vi "decode_serial_string.vi"(8 "Error In":errorcluster, 11 "Input Str":string) -> (0 "Error Out":errorcluster, 2 "Time":dbl, 3 "Current Values":T1)   [LabVIEW 2019]
doc: "Decode the serial string into its components."
uses:
  current_values_cluster_typedef.ctl
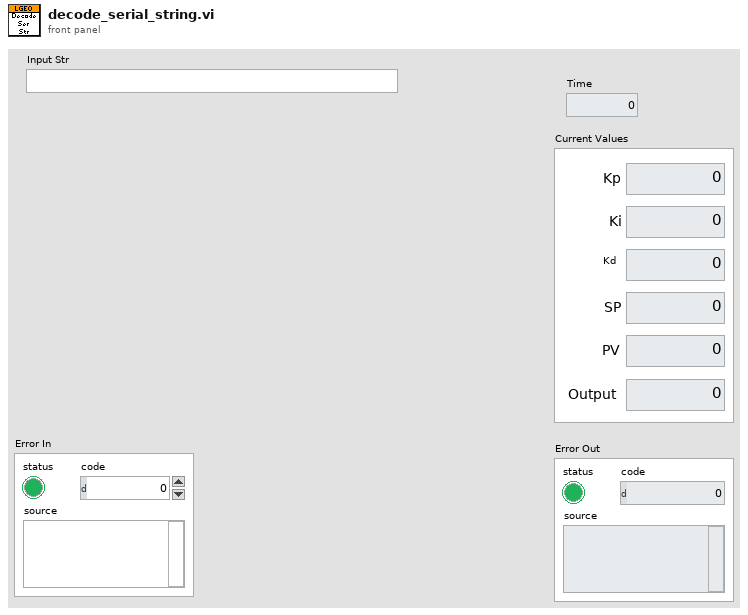
[diagram p1: front panel]
types:
  T1 = typedef "current_values_cluster_typedef.ctl" = cluster{"Kp":dbl, "Ki":dbl, "Kd":dbl, "SP":dbl, "PV":dbl, "Output":dbl}
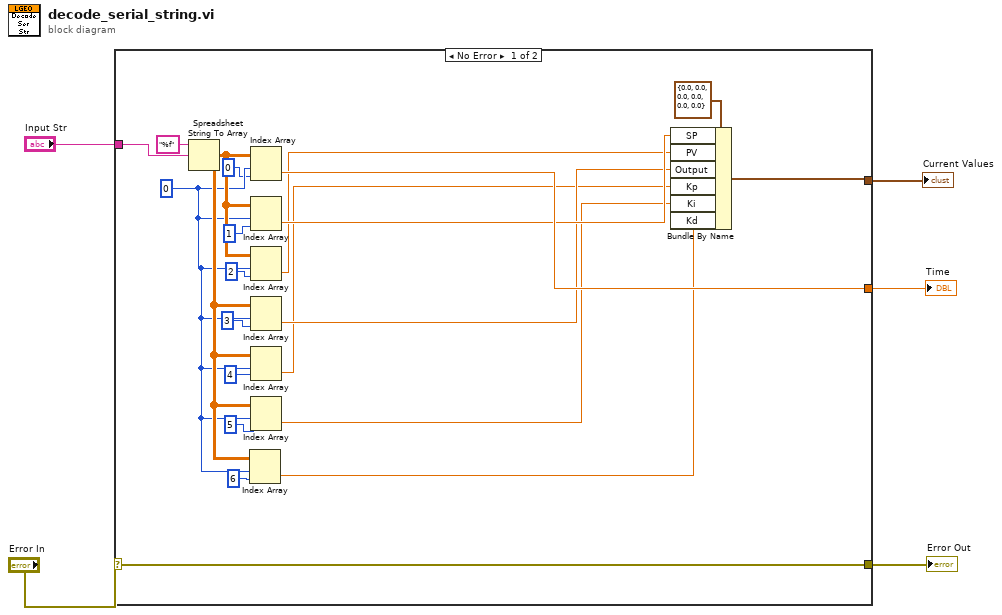
[diagram p0: block diagram]
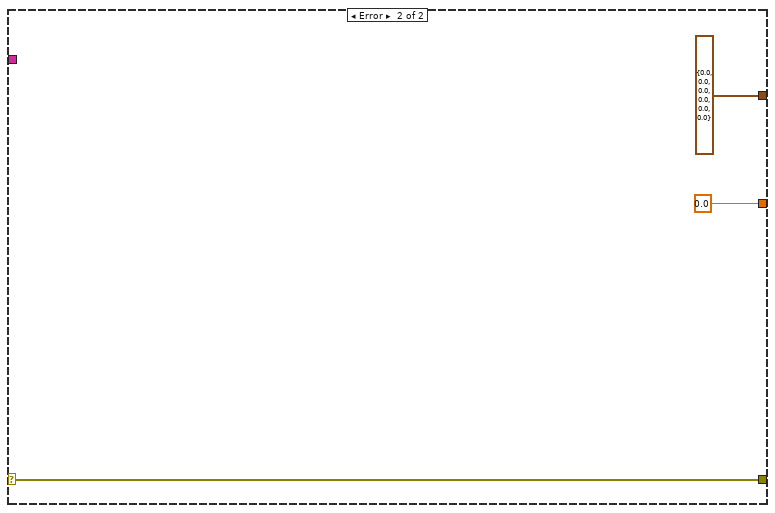
[diagram p2: hidden frame]
diagram:
  n1 = case shown="No Error" "Error In" {
    selector: "Error In" -> [w24 w29]
    tunnel: [w24 w29] -> w4
    tunnel: [w22 T1 {"Kp"=0.0, "Ki"=0.0, "Kd"=0.0, "SP"=0.0, "PV"=0.0, "Output"=0.0} ("Current Values")] -> w3
    tunnel: [w21 0.0 ("Time")] -> w2
    tunnel: "Input Str" -> [w26 _]
    frame No Error {
      w13 = 0
      n2 = Spreadsheet String To Array(format string="%f", spreadsheet string=w26) -> (array=w17:dbl[][])  [unwired: 2 in]
      n3 = Index Array(array=w17, index (row)=w13, index (col)=6) -> (element=w16:dbl)
      n4 = Index Array(array=w17, index (row)=w13, index (col)=0) -> (element=w21:dbl)
      n5 = Index Array(array=w17, index (row)=w13, index (col)=1) -> (element=w20:dbl)
      n6 = Index Array(array=w17, index (row)=w13, index (col)=2) -> (element=w19:dbl)
      n7 = Index Array(array=w17, index (row)=w13, index (col)=3) -> (element=w18:dbl)
      n8 = Index Array(array=w17, index (row)=w13, index (col)=4) -> (element=w14:dbl)
      n9 = Index Array(array=w17, index (row)=w13, index (col)=5) -> (element=w15:dbl)
      n10 = Bundle By Name(cluster=T1 {"Kp"=0.0, "Ki"=0.0, "Kd"=0.0, "SP"=0.0, "PV"=0.0, "Output"=0.0} ("Current Values"), "SP"=w20, "PV"=w19, "Output"=w18, "Kp"=w14, "Ki"=w15, "Kd"=w16) -> (w22:T1)
    }
    frame Error {
    }
  }
  "Current Values" <- w3
  "Error Out" <- w4
  "Time" <- w2
